vi "Layout.vi"(0 "reference":refnum<class "StateTransitionEdge.lvclass">, 1 "graph":refnum<class "Graph.lvclass">, 2 "graphics":refnum<class "Graphics.lvclass">, 3 "grid":refnum<class "Grid.lvclass">, 5 "error in (no error)":errorcluster) -> (14 "reference out":refnum<class "StateTransitionEdge.lvclass">, 19 "error out":errorcluster)   [LabVIEW 2016, in "StateTransitionEdge.lvclass"]
doc: "Layout"
uses:
  <resource>/Framework/Providers/Open_GDS/UML/StateTransitionEdge_class/StateTransitionEdge.lvclass
  C:/Program Files (x86)/National Instruments/LabVIEW 2016/resource/Framework/Providers/Open_GDS/UML/ClassRelationshipEdge_class/ClassRelationshipEdge.lvclass
  <resource>/Framework/Providers/Open_GDS/UML/Grid_class/Grid.lvclass
  <resource>/Framework/Providers/Open_GDS/UML/Graphics_class/Graphics.lvclass
  <resource>/Framework/Providers/Open_GDS/UML/Graph_class/Graph.lvclass
  <resource>/Framework/Providers/Open_GDS/UML/BentStyle_class/BentStyle.lvclass
  <resource>/Framework/Providers/Open_GDS/UML/ClassRelationshipEdge_class/ClassRelationshipEdge.lvclass
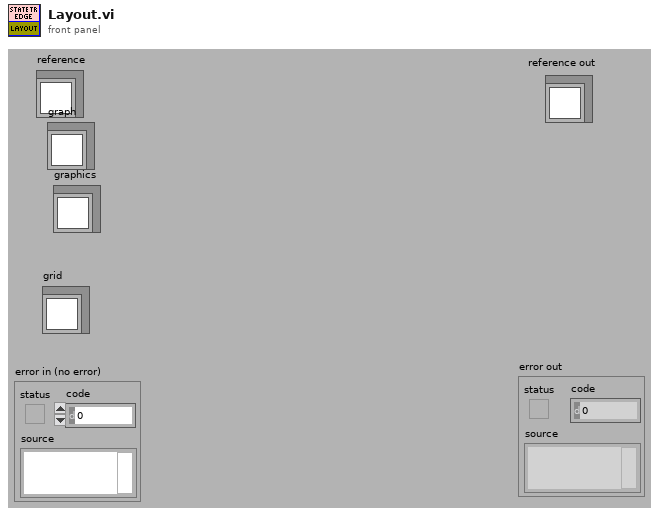
[diagram p1: front panel]
types:
  T1 = typedef "ClassRelationshipEdge.lvclass/ObjectAttributes.ctl" = cluster{"bentStyleRef":refnum<class "BentStyle.lvclass">, "startConnectionOffset":cluster{"x":i32, "y":i32}, "endConnectionOffset":cluster{"x":i32, "y":i32}, "MidLineOffset":cluster{"x":i32, "y":i32}, "DepClass":T2}
  T2 = typedef "ReversedEngineering_ViDependencyDetailsType.ctl" = cluster{"ThisVIs/Ctls":path[], "Dependent_VIs/Ctls":path[]}
  T3 = typedef "BentStyle.lvclass/BentStyleType.ctl" = enum16{"STRAIGHT", "HV", "VH", "HVH", "VHV", "ARC"}
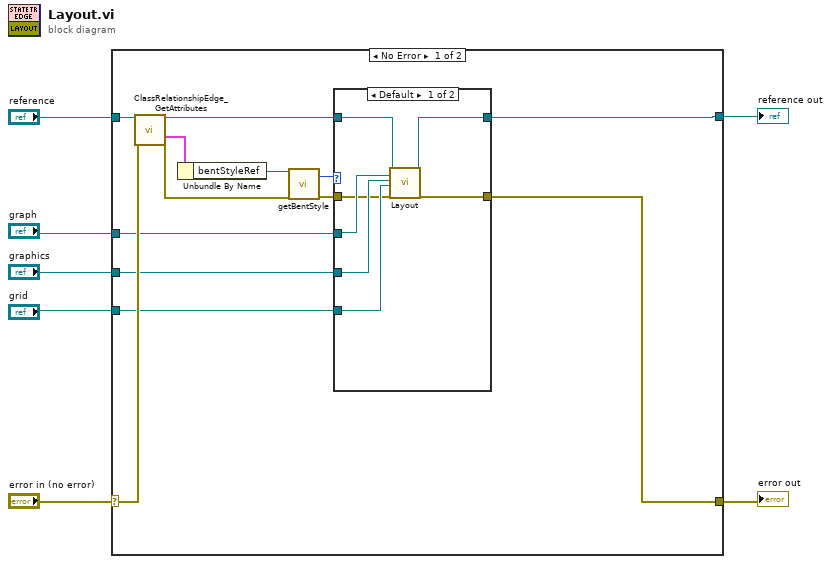
[diagram p0: block diagram]
diagram:
  n1 = case shown="No Error" "error in (no error)" {
    selector: "error in (no error)" -> [w20 w30]
    tunnel: "reference" -> [w19 w31]
    tunnel: [w10 w30] -> w5
    tunnel: [w9 w31] -> w4
    tunnel: "graph" -> [w14 _]
    tunnel: "graphics" -> [w13 _]
    tunnel: "grid" -> [w12 _]
    frame No Error {
      n2 = call <resource>:"ClassRelationshipEdge_GetAttributes.vi"("reference in"=w19, "error in (no error)"=w20) -> ("reference out"=w15:refnum<class "StateTransitionEdge.lvclass">, "Data"=w8:T1, "error out"=w11:errorcluster)  [unwired: 14 in, 1 out]
      n3 = Unbundle By Name(w8) -> ("bentStyleRef"=w18:refnum<class "BentStyle.lvclass">)
      n4 = call-dynamic "getBentStyle.vi"("reference"=w18, "error in (no error)"=w11) -> ("bentStyle"=w17:T3, "error out"=w16:errorcluster)  [unwired: 15 in, 1 out]
      n5 = case shown="Default" w17 {
        tunnel: w16 -> [w23 w29]
        tunnel: w15 -> [w27 w28]
        tunnel: w14 -> [w26 _]
        tunnel: w13 -> [w25 _]
        tunnel: w12 -> [w24 _]
        tunnel: [w22 w29] -> w10
        tunnel: [w21 w28] -> w9
        frame Default {
          n6 = call-parent "Layout.vi"("reference"=w27, "graph"=w26, "graphics"=w25, "grid"=w24, "error in (no error)"=w23) -> ("reference out"=w21:refnum<class "StateTransitionEdge.lvclass">, "error out"=w22:errorcluster)  [unwired: 13 in]
        }
        frame "ARC" {
        }
      }
    }
    frame Error {
    }
  }
  "reference out" <- w4
  "error out" <- w5
